vi "myDAQ Errors.vi"(8 "error in (no error)":errorcluster) -> (0 "error out":errorcluster)   [LabVIEW 2014]
doc: "This VI is designed to handel common myDAQ errors and give more useful specific error dialogs. It also finds a control names \"Stop\" in the calling VI and toggels it true to stop the VI."
uses:
  <vilib>/regexp/Match Regular Expression.xnode
panel:
  out "call chain":string[](array[string])
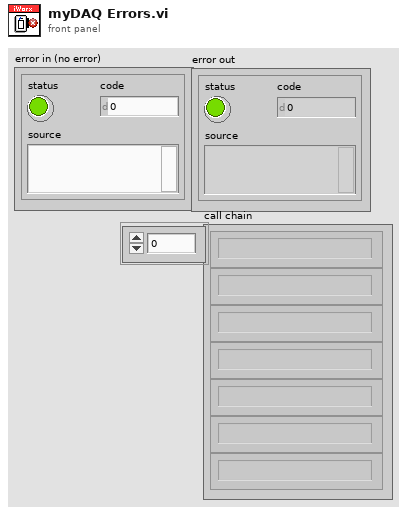
[diagram p1: front panel]
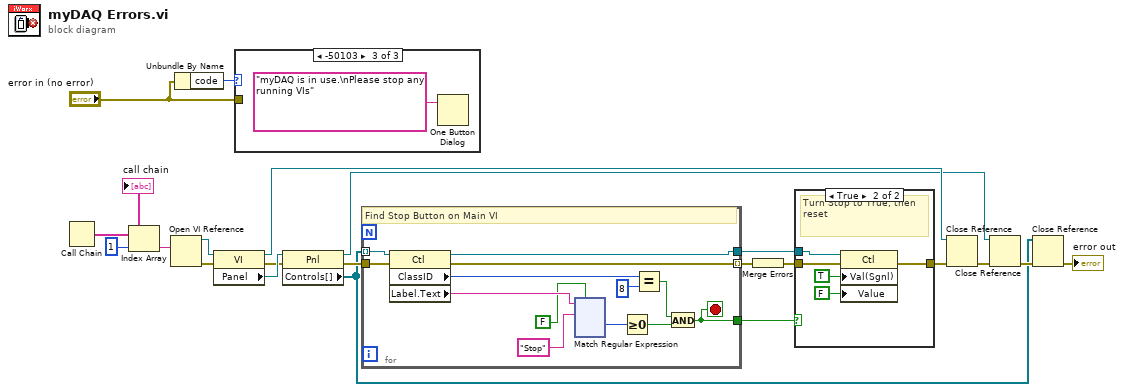
[diagram p0: block diagram]
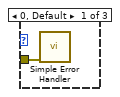
[diagram p3: hidden frame]
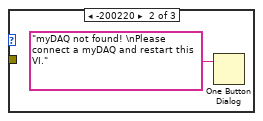
[diagram p4: hidden frame]
diagram:
  n1 = Call Chain() -> (call chain=w20:string[])
  "call chain" <- w20
  n2 = Index Array(array=w20, index=1) -> (element=w18:string)
  n3 = Open VI Reference(vi path=w18) -> (vi reference=w17:refnum<vi>, error out=w16:errorcluster)  [unwired: 5 in]
  n4 = Unbundle By Name("error in (no error)") -> ("code"=w21:i32)
  n5 = property class="VI"(reference=w17, error in=w16) -> (reference out=w8:refnum<vi>, error out=w11:errorcluster, "Panel"=w15:refnum<vi>)
  n6 = case shown="-50103" w21 {
    tunnel: "error in (no error)" -> [w22 _ _]
    frame 0, Default {
      n7 = call <vilib>:"Simple Error Handler.vi"("error in (no error)"=w22) -> ()  [unwired: 4 in, 5 out]
    }
    frame -200220 {
      n8 = One Button Dialog(message="myDAQ not found! \nPlease connect a myDAQ and restart this VI.") -> ()  [unwired: 1 in, 1 out]
    }
    frame -50103 {
      n9 = One Button Dialog(message="myDAQ is in use.\nPlease stop any running VIs") -> ()  [unwired: 1 in, 1 out]
    }
  }
  n10 = property class="Pnl"(reference=w15, error in=w11) -> (reference out=w5:refnum<vi>, error out=w12:errorcluster, "Controls[]"=w3:refnum<vi>[])
  n11 = for {
    tunnel: w3 -> [w37] mode=indexing
    tunnel: [w33] -> w14
    tunnel: [w32] -> w13
    tunnel: [w31] -> w10 mode=indexing
    tunnel: w12 -> [w30]
    stop <- w32 stop-if-true
    # "Find Stop Button on Main VI"
    n12 = property class="Ctl"(reference=w37, error in=w30) -> (reference out=w33:refnum<vi>, error out=w31:errorcluster, "ClassID"=w36:u32, "Label.Text"=w29:string)
    n13 = xnode "Match Regular Expression"("input string"=w29, "regular expression"="Stop" ("y"), "ignore case? (F)"=FALSE) -> ("offset past match"=w26:i32)  [unwired: 3 in, 4 out]
    n14 = Greater Or Equal To 0?(x=w26) -> (x >= 0?=w25:bool)
    n15 = Equal?(x=w36, y=u32 8) -> (x = y?=w34:bool)
    n16 = And(x=w34, y=w25) -> (x .and. y?=w32:bool)
  }
  n17 = Merge Errors(w10) -> (w9:errorcluster)
  n18 = case shown="True" w13 {
    tunnel: w14 -> [_ w154]
    tunnel: w9 -> [w149 w152]
    tunnel: [w149 w150] -> w7
    frame False {
      # "Do nothing"
    }
    frame True {
      # "Turn Stop to True, then reset"
      n19 = property class="Ctl"(reference=w154, error in=w152, "Val(Sgnl)"=TRUE, "Value"=FALSE) -> (error out=w150:errorcluster)  [unwired: 1 out]
    }
  }
  n20 = Close Reference(reference=w8, error in (no error)=w7) -> (error out=w6:errorcluster)
  n21 = Close Reference(reference=w5, error in (no error)=w6) -> (error out=w4:errorcluster)
  n22 = Close Reference(reference=w3, error in (no error)=w4) -> (error out=→"error out":errorcluster)
